vi "Get Instance VI Path.vi"(1 "instVIref":T1, 2 "diagram":refnum<vi>) -> (0 "instance path":path)   [LabVIEW 2020, in "NI_TargetHelper.lvlib"]
uses:
  <vilib>/TargetSupport/NI_TargetHelper/NI_TargetHelper.lvlib
  <vilib>/TargetSupport/NI_TargetHelper/Instance VIref.ctl
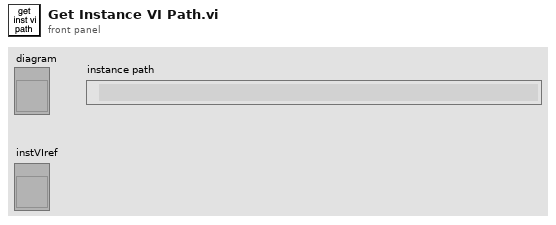
[diagram p1: front panel]
types:
  T1 = typedef "NI_TargetHelper.lvlib/Instance VIref.ctl" = refnum<vi>
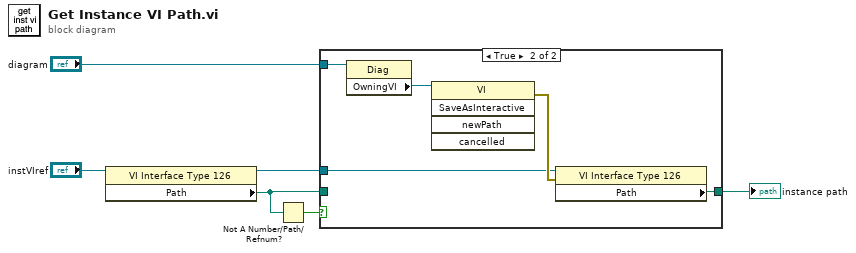
[diagram p0: block diagram]
diagram:
  n1 = property class="VI Interface Type 126"(reference="instVIref") -> (reference out=w5:T1, "Path"=w4:path)  [unwired: 1 in, 1 out]
  n2 = Not A Number/Path/Refnum?(number/path/refnum=w4) -> (NaN/Path/Refnum?=w6:bool)
  n3 = case shown="True" w6 {
    tunnel: "diagram" -> [_ w12]
    tunnel: w5 -> [_ w9]
    tunnel: [w7 w8] -> w1
    tunnel: w4 -> [w7 _]
    frame False {
    }
    frame True {
      n4 = property class="Diag"(reference=w12) -> ("OwningVI"=w11:refnum<vi>)  [unwired: 1 in, 2 out]
      n5 = invoke class="VI" method="SaveAsInteractive"(reference=w11) -> (error out=w10:errorcluster)  [unwired: 4 in, 4 out]
      n6 = property class="VI Interface Type 126"(reference=w9, error in=w10) -> ("Path"=w8:path)  [unwired: 2 out]
    }
  }
  "instance path" <- w1
